vi "Write METADATA.vi"(8 "error in (no error)":errorcluster, 10 "METADATA":variant, 11 "CubeLogger in":refnum<class "CubeLogger.lvclass">) -> (0 "error out":errorcluster, 3 "CubeLogger out":refnum<class "CubeLogger.lvclass">)   [LabVIEW 2018, in "CubeLogger.lvclass"]
uses:
  CubeLogger.lvclass
  CubeLogger.lvclass/CubeLogger.ctl
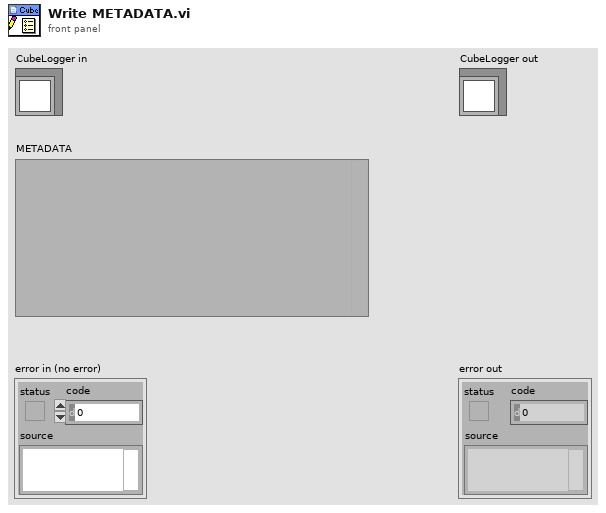
[diagram p1: front panel]
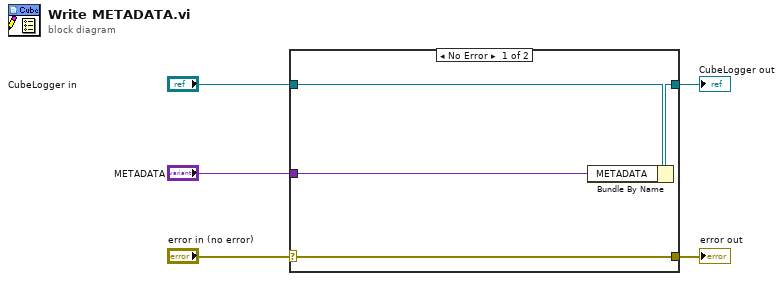
[diagram p0: block diagram]
diagram:
  n1 = case shown="No Error" "error in (no error)" {
    selector: "error in (no error)" -> [w9 w10]
    tunnel: [w9 w10] -> w4
    tunnel: [w7 w11] -> w2
    tunnel: "CubeLogger in" -> [w8 w11]
    tunnel: "METADATA" -> [w6 _]
    frame No Error {
      n2 = Bundle By Name(cluster=w8, "METADATA"=w6) -> (w7:refnum<class "CubeLogger.lvclass">)
    }
    frame Error {
    }
  }
  "error out" <- w4
  "CubeLogger out" <- w2
